vi "Set Value of LabVIEW Base Type.vi"(8 "error in (no error)":errorcluster, 10 "LabVIEW Base Type":refnum<vi>, 11 "JSON Tree Node":variant) -> (0 "error out":errorcluster)   [LabVIEW 2013, in "i3-json.lvlib"]
doc: "This VI takes a JSON Node (all types besides JSON Object) and assigns the value to the LabVIEW Base Type of compatible reference.\n\nIf the LabVIEW base type is an array of boolean, numeric, or string this function will attempt to check if a JSON Array type will map"
uses:
  i3-json.lvlib
  JSON Types/JSON Type.ctl
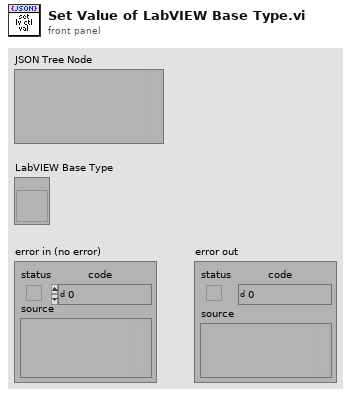
[diagram p1: front panel]
types:
  T1 = typedef "i3-json.lvlib/JSON Type.ctl" = enum8{"JSON Compatible", "JSON Array", "JSON Object", "JSON Null", "Double", "String", "Boolean", "Unknown"}
  T2 = enum8{"Invalid Type", "Void", "I8", "I16", "I32", "I64", "U8", "U16", "U32", "U64", "Single Float", "Double Float", "Extended Float", "Single Complex", "Double Complex", "Extended Complex", "Enum U8", "Enum U16", "Enum U32", "Enum U64", "Single Float With Unit", "Double Float With Unit", "Extended Float With Unit", "Single Complex with Unit", "Double Complex with Unit", "Extended Complex with Unit", "Boolean", "String", "Path", "Picture", "Tag", "Array", "Cluster", "Variant", "LV Variant", "Waveform", "Timestamp", "Digital Waveform", "Digital Data", "ExpressData", "Refnum", "External Data", "VI", "Poly VI", "LabVIEW Class Instance", "Fixed Point"}
  T3 = typedef "i3-json.lvlib/JSON Compatible Type.ctl" = enum16{"1D Double Array", "1D String Array", "1D Boolean Array", "Unknown"}
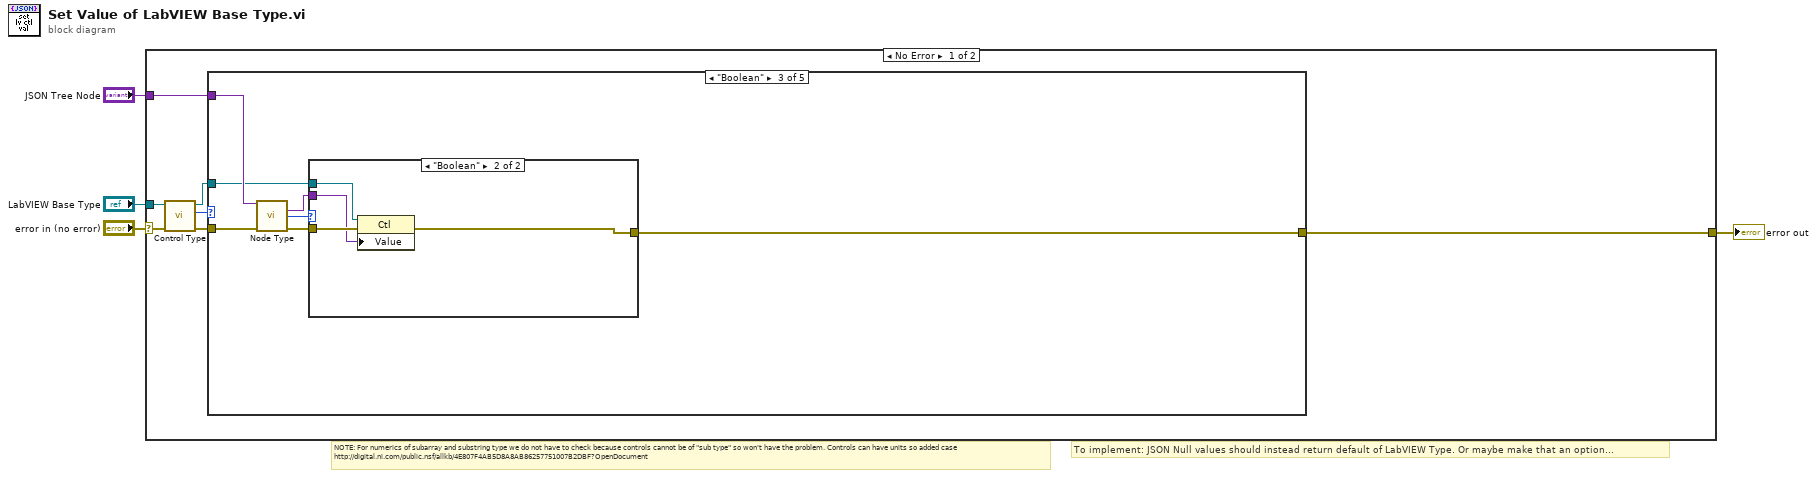
[diagram p0: block diagram]
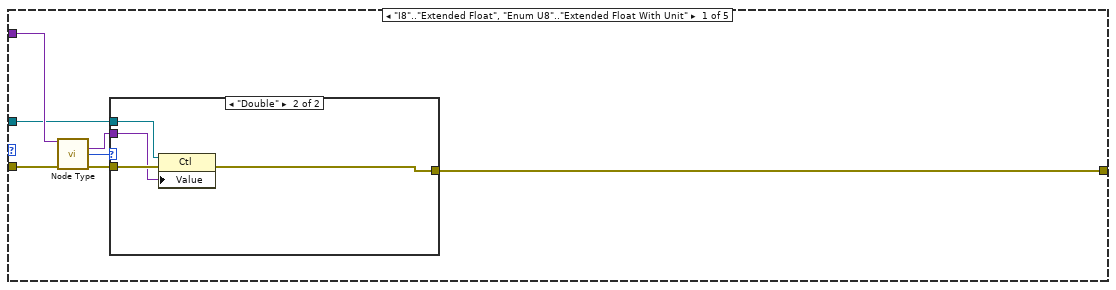
[diagram p2: hidden frame]
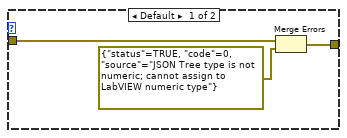
[diagram p3: hidden frame]
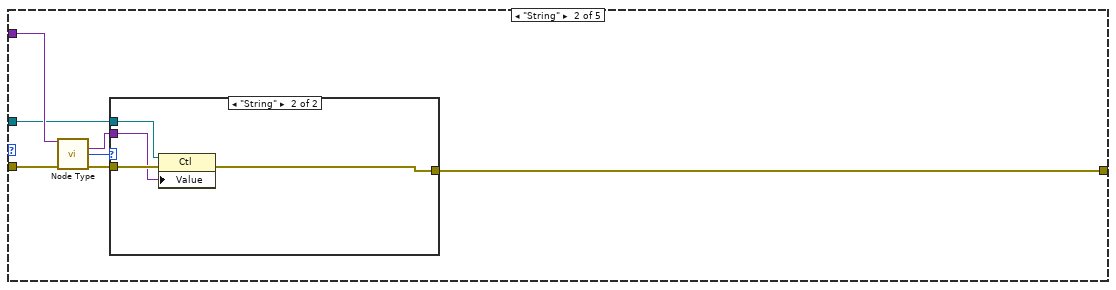
[diagram p4: hidden frame]
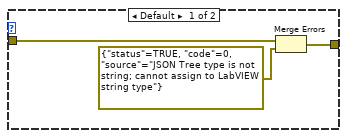
[diagram p5: hidden frame]
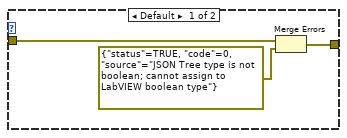
[diagram p6: hidden frame]
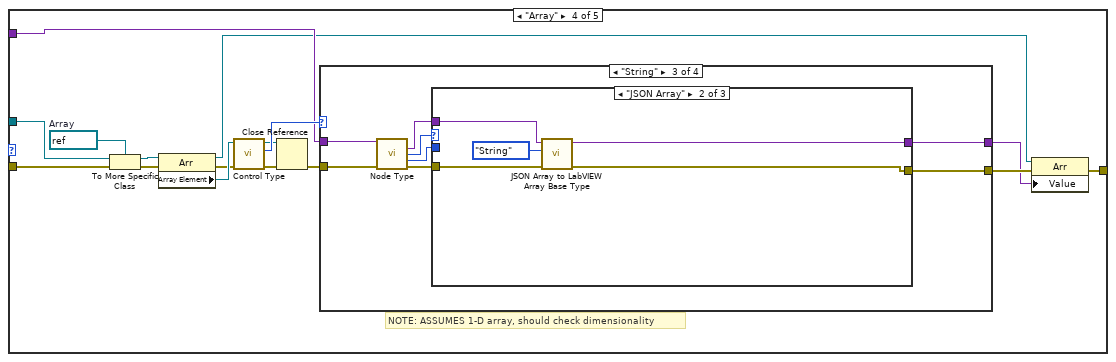
[diagram p7: hidden frame]
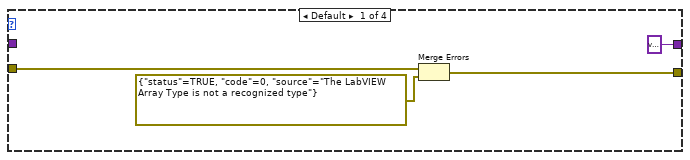
[diagram p8: hidden frame]
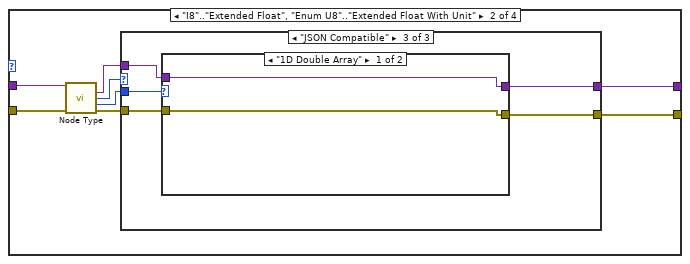
[diagram p9: hidden frame]
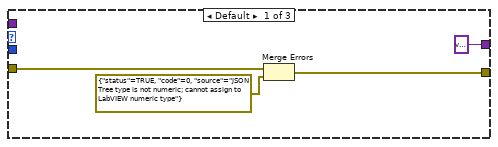
[diagram p10: hidden frame]
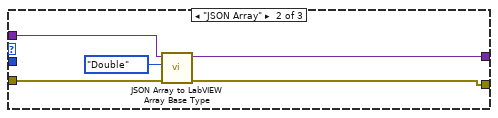
[diagram p11: hidden frame]
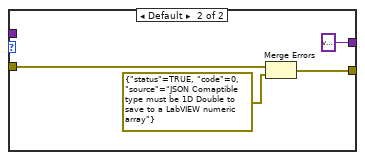
[diagram p12: hidden frame]
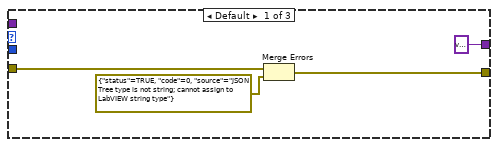
[diagram p13: hidden frame]
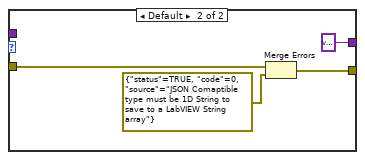
[diagram p15: hidden frame]
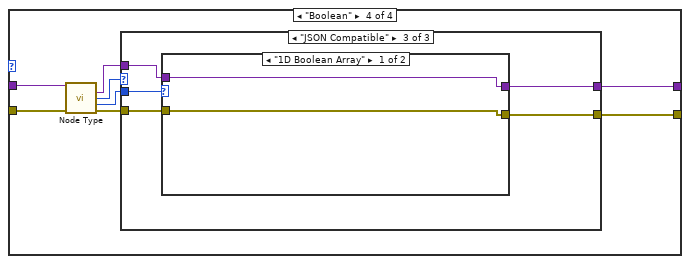
[diagram p16: hidden frame]
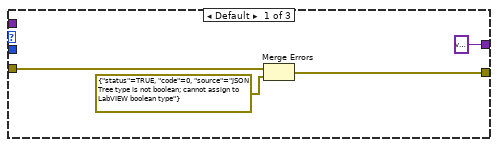
[diagram p17: hidden frame]
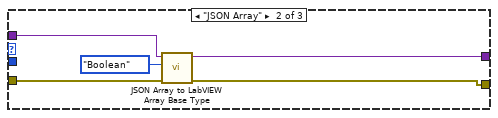
[diagram p18: hidden frame]
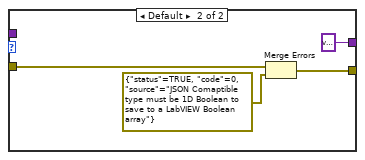
[diagram p19: hidden frame]
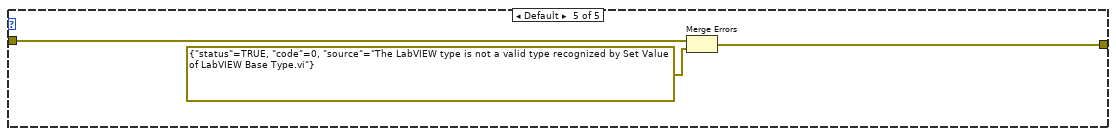
[diagram p20: hidden frame]
diagram:
  # "NOTE: For numerics of subarray and substring type we do not have to check because controls cannot be of \"sub type\" so won't have the problem. Controls can have units so added case\nhttp://digital.ni.com/public.nsf/allkb/4E807F4AB5D8A8AB86257751007B2DBF?OpenDocument"
  # "To implement: JSON Null values should instead return default of LabVIEW Type. Or maybe make that an option..."
  n1 = case shown="No Error" "error in (no error)" {
    selector: "error in (no error)" -> [w11 w161]
    tunnel: "LabVIEW Base Type" -> [w10 _]
    tunnel: "JSON Tree Node" -> [w7 _]
    tunnel: [w5 w161] -> w1
    frame No Error {
      n2 = call "Control Type.vi"("error in (no error)"=w11, "Control in"=w10) -> ("error out"=w6:errorcluster, "Type"=w9:T2, "Control out"=w8:refnum<vi>)  [unwired: 7 in]
      n3 = case shown="\"Boolean\"" w9 {
        tunnel: w8 -> [w13 w27 w41 w68 _]
        tunnel: w7 -> [w18 w32 w46 w63 _]
        tunnel: w6 -> [w17 w31 w45 w69 w160]
        tunnel: [w12 w26 w40 w60 w159] -> w5
        frame "I8".."Extended Float", "Enum U8".."Extended Float With Unit" {
          n4 = call "Node Type.vi"("JSON Tree In"=w18, "error in (no error)"=w17) -> ("Value"=w14:variant, "JSON Type"=w16:T1, "error out"=w15:errorcluster)  [unwired: 9 in, 2 out]
          n5 = case shown="\"Double\"" w16 {
            tunnel: w15 -> [w21 w25]
            tunnel: [w19 w22] -> w12
            tunnel: w14 -> [_ w24]
            tunnel: w13 -> [_ w23]
            frame Default {
              n6 = Merge Errors(w21, errorcluster {"status"=TRUE, "code"=0, "source"="JSON Tree type is not numeric; cannot assign to LabVIEW numeric type"} ("error in")) -> (w19:errorcluster)
            }
            frame "Double" {
              n7 = property class="Ctl"(reference=w23, error in=w25, "Value"=w24) -> (error out=w22:errorcluster)  [unwired: 1 out]
            }
          }
        }
        frame "String" {
          n8 = call "Node Type.vi"("JSON Tree In"=w32, "error in (no error)"=w31) -> ("Value"=w28:variant, "JSON Type"=w30:T1, "error out"=w29:errorcluster)  [unwired: 9 in, 2 out]
          n9 = case shown="\"String\"" w30 {
            tunnel: w29 -> [w35 w39]
            tunnel: [w33 w36] -> w26
            tunnel: w28 -> [_ w38]
            tunnel: w27 -> [_ w37]
            frame Default {
              n10 = Merge Errors(w35, errorcluster {"status"=TRUE, "code"=0, "source"="JSON Tree type is not string; cannot assign to LabVIEW string type"} ("error in")) -> (w33:errorcluster)
            }
            frame "String" {
              n11 = property class="Ctl"(reference=w37, error in=w39, "Value"=w38) -> (error out=w36:errorcluster)  [unwired: 1 out]
            }
          }
        }
        frame "Boolean" {
          n12 = call "Node Type.vi"("JSON Tree In"=w46, "error in (no error)"=w45) -> ("Value"=w42:variant, "JSON Type"=w44:T1, "error out"=w43:errorcluster)  [unwired: 9 in, 2 out]
          n13 = case shown="\"Boolean\"" w44 {
            tunnel: w43 -> [w49 w53]
            tunnel: [w47 w50] -> w40
            tunnel: w42 -> [_ w52]
            tunnel: w41 -> [_ w51]
            frame Default {
              n14 = Merge Errors(w49, errorcluster {"status"=TRUE, "code"=0, "source"="JSON Tree type is not boolean; cannot assign to LabVIEW boolean type"} ("error in")) -> (w47:errorcluster)
            }
            frame "Boolean" {
              n15 = property class="Ctl"(reference=w51, error in=w53, "Value"=w52) -> (error out=w50:errorcluster)  [unwired: 1 out]
            }
          }
        }
        frame "Array" {
          w62 = refnum<vi> refnum  # Array
          # "NOTE: ASSUMES 1-D array, should check dimensionality"
          n16 = To More Specific Class(target class=w62, reference=w68, error in=w69) -> (specific class reference=w59:refnum<vi>, error out=w67:errorcluster)
          n17 = property class="Arr"(reference=w59, error in=w67) -> (reference out=w54:refnum<vi>, error out=w65:errorcluster, "Array Element"=w66:refnum<vi>)
          n18 = call "Control Type.vi"("error in (no error)"=w65, "Control in"=w66) -> ("error out"=w57:errorcluster, "Type"=w64:T2, "Control out"=w55:refnum<vi>)  [unwired: 7 in]
          n19 = Close Reference(reference=w55, error in (no error)=w57) -> (error out=w56:errorcluster)
          n20 = case shown="\"String\"" w64 {
            tunnel: w56 -> [w73 w79 w107 w135]
            tunnel: w63 -> [_ w78 w106 w134]
            tunnel: [w71 w75 w103 w131] -> w61
            tunnel: [variant ("Value") w74 w102 w130] -> w58
            frame Default {
              n21 = Merge Errors(w73, errorcluster {"status"=TRUE, "code"=0, "source"="The LabVIEW Array Type is not a recognized type"} ("error in")) -> (w71:errorcluster)
            }
            frame "I8".."Extended Float", "Enum U8".."Extended Float With Unit" {
              n22 = call "Node Type.vi"("JSON Tree In"=w78, "error in (no error)"=w79) -> ("Value"=w81:variant, "JSON Type"=w77:T1, "JSON Compatible Type"=w76:T3, "error out"=w80:errorcluster)  [unwired: 9 in, 1 out]
              n23 = case shown="\"JSON Compatible\"" w77 {
                tunnel: w80 -> [w85 w90 w94]
                tunnel: w81 -> [_ w89 w93]
                tunnel: [w83 w87 w95] -> w75
                tunnel: w76 -> [_ _ w92]
                tunnel: [variant ("Value") w86 w91] -> w74
                frame Default {
                  n24 = Merge Errors(w85, errorcluster {"status"=TRUE, "code"=0, "source"="JSON Tree type is not numeric; cannot assign to LabVIEW numeric type"} ("error in")) -> (w83:errorcluster)
                }
                frame "JSON Array" {
                  n25 = call "JSON Array to LabVIEW Array Base Type.vi"("error in (no error)"=w90, "Type of Array In"=JSON_Type."Double", "JSON Array In"=w89) -> ("error out"=w87:errorcluster, "LabVIEW Array Base Type Out"=w86:variant)  [unwired: 7 in]
                }
                frame "JSON Compatible" {
                  n26 = case shown="\"1D Double Array\"" w92 {
                    tunnel: w94 -> [w96 w101]
                    tunnel: [w96 w100] -> w95
                    tunnel: w93 -> [w97 _]
                    tunnel: [w97 variant ("Value")] -> w91
                    frame "1D Double Array" {
                    }
                    frame Default {
                      n27 = Merge Errors(w101, errorcluster {"status"=TRUE, "code"=0, "source"="JSON Comaptible type must be 1D Double to save to a LabVIEW numeric array"} ("error in (no error)")) -> (w100:errorcluster)
                    }
                  }
                }
              }
            }
            frame "String" {
              n28 = call "Node Type.vi"("JSON Tree In"=w106, "error in (no error)"=w107) -> ("Value"=w109:variant, "JSON Type"=w105:T1, "JSON Compatible Type"=w104:T3, "error out"=w108:errorcluster)  [unwired: 9 in, 1 out]
              n29 = case shown="\"JSON Array\"" w105 {
                tunnel: w108 -> [w113 w118 w122]
                tunnel: w109 -> [_ w117 w121]
                tunnel: [w111 w115 w123] -> w103
                tunnel: w104 -> [_ _ w120]
                tunnel: [variant ("Value") w114 w119] -> w102
                frame Default {
                  n30 = Merge Errors(w113, errorcluster {"status"=TRUE, "code"=0, "source"="JSON Tree type is not string; cannot assign to LabVIEW string type"} ("error in")) -> (w111:errorcluster)
                }
                frame "JSON Array" {
                  n31 = call "JSON Array to LabVIEW Array Base Type.vi"("error in (no error)"=w118, "Type of Array In"=JSON_Type."String", "JSON Array In"=w117) -> ("error out"=w115:errorcluster, "LabVIEW Array Base Type Out"=w114:variant)  [unwired: 7 in]
                }
                frame "JSON Compatible" {
                  n32 = case shown="\"1D String Array\"" w120 {
                    tunnel: w122 -> [w124 w129]
                    tunnel: [w124 w128] -> w123
                    tunnel: w121 -> [w125 _]
                    tunnel: [w125 variant ("Value")] -> w119
                    frame "1D String Array" {
                    }
                    frame Default {
                      n33 = Merge Errors(w129, errorcluster {"status"=TRUE, "code"=0, "source"="JSON Comaptible type must be 1D String to save to a LabVIEW String array"} ("error in (no error)")) -> (w128:errorcluster)
                    }
                  }
                }
              }
            }
            frame "Boolean" {
              n34 = call "Node Type.vi"("JSON Tree In"=w134, "error in (no error)"=w135) -> ("Value"=w137:variant, "JSON Type"=w133:T1, "JSON Compatible Type"=w132:T3, "error out"=w136:errorcluster)  [unwired: 9 in, 1 out]
              n35 = case shown="\"JSON Compatible\"" w133 {
                tunnel: w136 -> [w141 w146 w150]
                tunnel: w137 -> [_ w145 w149]
                tunnel: [w139 w143 w151] -> w131
                tunnel: w132 -> [_ _ w148]
                tunnel: [variant ("Value") w142 w147] -> w130
                frame Default {
                  n36 = Merge Errors(w141, errorcluster {"status"=TRUE, "code"=0, "source"="JSON Tree type is not boolean; cannot assign to LabVIEW boolean type"} ("error in")) -> (w139:errorcluster)
                }
                frame "JSON Array" {
                  n37 = call "JSON Array to LabVIEW Array Base Type.vi"("error in (no error)"=w146, "Type of Array In"=JSON_Type."Boolean", "JSON Array In"=w145) -> ("error out"=w143:errorcluster, "LabVIEW Array Base Type Out"=w142:variant)  [unwired: 7 in]
                }
                frame "JSON Compatible" {
                  n38 = case shown="\"1D Boolean Array\"" w148 {
                    tunnel: w150 -> [w152 w157]
                    tunnel: [w152 w156] -> w151
                    tunnel: w149 -> [w153 _]
                    tunnel: [w153 variant ("Value")] -> w147
                    frame "1D Boolean Array" {
                    }
                    frame Default {
                      n39 = Merge Errors(w157, errorcluster {"status"=TRUE, "code"=0, "source"="JSON Comaptible type must be 1D Boolean to save to a LabVIEW Boolean array"} ("error in (no error)")) -> (w156:errorcluster)
                    }
                  }
                }
              }
            }
          }
          n40 = property class="Arr"(reference=w54, error in=w61, "Value"=w58) -> (error out=w60:errorcluster)  [unwired: 1 out]
        }
        frame Default {
          n41 = Merge Errors(w160, errorcluster {"status"=TRUE, "code"=0, "source"="The LabVIEW type is not a valid type recognized by Set Value of LabVIEW Base Type.vi"} ("error in")) -> (w159:errorcluster)
        }
      }
    }
    frame Error {
    }
  }
  "error out" <- w1
